vi "Result_Test.vi"(8 "error in (no error)":errorcluster caption="entrée d'erreur (pas d'erreur)", 11 "Get_Voltage en entrée":refnum<class "Read_Saturation_LED.lvclass">) -> (0 "error out":errorcluster caption="sortie d'erreur", 3 "Get_Voltage en sortie":refnum<class "Read_Saturation_LED.lvclass">)   [LabVIEW 2020, in "Library Test.lvlib" / "Read_Saturation_LED.lvclass"]
uses:
  Read_Saturation_LED.lvclass
  C:/Users/ngarcin/OneDrive - Altyor/Standard TB/Class/Test/Test (Default)/Test (Default).lvclass
  JSON API/JSON Value/Set from JSON string.vi
  Instrument/Instrument (Default)/Class Instrument (Default).lvclass
  JSON API/JSON Value/JSON Value.lvclass
  Read_Led_Analyser/Read_Led_Analyser.lvclass
  Read_Saturation_LED.lvclass/Read_Saturation_LED.ctl
  JSON API/Variant JSON/Variant JSON.lvlib
  JSON API/Get Polymorphic/JSON GetSet.lvlib
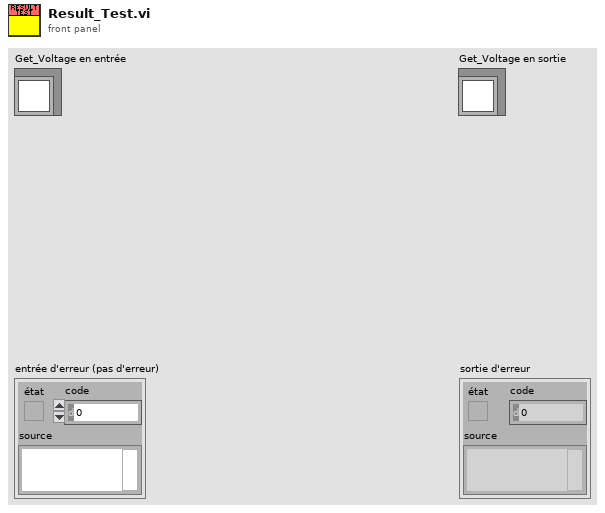
[diagram p1: front panel]
types:
  T1 = cluster{"Hue":dbl, "Saturation":u32, "Intensity":u32}
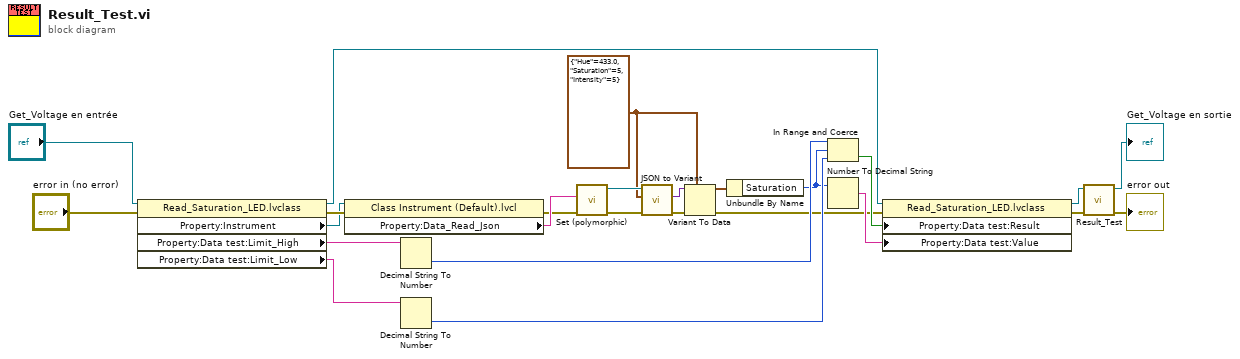
[diagram p0: block diagram]
diagram:
  w17 = T1 {"Hue"=433.0, "Saturation"=5, "Intensity"=5} ("Parameter")
  n1 = property class="Read_Saturation_LED.lvclass"(reference="Get_Voltage en entrée", error in="error in (no error)") -> (reference out=w14:refnum<class "Read_Saturation_LED.lvclass">, error out=w3:errorcluster, "Property:Instrument"=w1:refnum<class "Class Instrument (Default).lvclass">, "Property:Data test:Limit_High"=w12:string, "Property:Data test:Limit_Low"=w11:string)
  n2 = property class="Class Instrument (Default).lvcl"(reference=w1, error in=w3) -> (error out=w2:errorcluster, "Property:Data_Read_Json"=w4:string)  [unwired: 1 out]
  n3 = Decimal String To Number(string=w12) -> (number=w10:i32)  [unwired: 2 in, 1 out]
  n4 = Decimal String To Number(string=w11) -> (number=w9:i32)  [unwired: 2 in, 1 out]
  n5 = call-poly "Set (polymorphic).vi"("error in (no error)"=w2, "JSON stream"=w4) -> ("error out"=w21:errorcluster, "JSON Value out"=w19:refnum<class "JSON Value.lvclass">)  [unwired: 7 in, 1 out]
  n6 = call "JSON to Variant.vi"("error in (no error)"=w21, "Variant (Data Type)"=w17, "JSON Value"=w19) -> ("error out"=w20:errorcluster, "Variant out"=w18:variant)  [unwired: 7 in]
  n7 = Variant To Data(error in=w20, type=w17, Variant=w18) -> (data=w16:T1, error out=w5:errorcluster)
  n8 = Unbundle By Name(w16) -> ("Saturation"=w7:u32)
  n9 = In Range and Coerce(upper limit=w10, x=w7, lower limit=w9) -> (In Range?=w8:bool)  [unwired: 1 out]
  n10 = Number To Decimal String(number=w7) -> (decimal integer string=w6:string)  [unwired: 1 in]
  n11 = property class="Read_Saturation_LED.lvclass"(reference=w14, error in=w5, "Property:Data test:Result"=w8, "Property:Data test:Value"=w6) -> (reference out=w13:refnum<class "Read_Saturation_LED.lvclass">, error out=w15:errorcluster)
  n12 = call-parent "Result_Test.vi"("error in (no error)"=w15, "Get_Voltage en entrée"=w13) -> ("error out"=→"error out":errorcluster, "Get_Voltage en sortie"=→"Get_Voltage en sortie":refnum<class "Read_Saturation_LED.lvclass">)  [unwired: 8 in]
